vi "Get.vi"(11 "Double in":refnum<class "Double.lvclass">) -> (2 "Value":dbl)   [LabVIEW 2020, in "Conditu2.lvlib" / "Columns.lvlib" / "Double.lvclass"]
uses:
  Double.lvclass
  Double.lvclass/Double.ctl
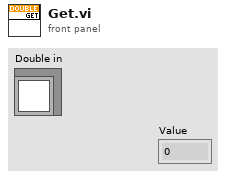
[diagram p1: front panel]
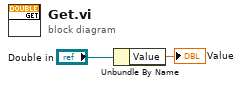
[diagram p0: block diagram]
diagram:
  n1 = Unbundle By Name("Double in") -> ("Value"=→"Value":dbl)
